vi "PCO_SetActiveRamSegment.vi"(8 "error in (no error)":errorcluster {"code" format="%x"}, 10 "wActSeg":u16, 11 "ph":u64) -> (0 "error out":errorcluster {"code" format="%x"}, 2 "ErrorMessage":i32 format="%x", 3 "ph out":u64)   [LabVIEW 2019, in "SDK.lvlib" / "StorageControl.lvlib"]
doc: "<b>Description:</b>\nThis function does set the active memory segment. Images from a subsequent recording are stored in the memory of the active segment. Relevant settings of the recorded images are also stored for each segment see also PCO_GetSegmentImageSettings.\nThis command will be rejected, if Recording State is [run], see PCO_GetRecordingState.\n\n<b>Supported camera type:</b>\npco.dimax, pco.1200, pco.1600, pco.2000, pco.4000\n\n<b>Descriptor dependency:</b>\ndwGeneralCapsDESC1: NO_RECORDER"
uses:
  StorageControl.lvlib
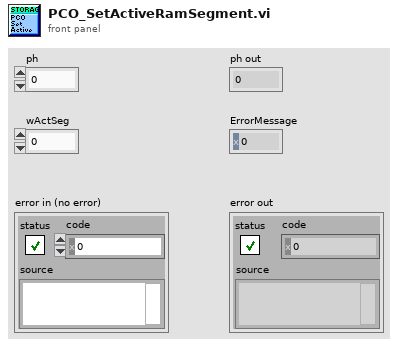
[diagram p1: front panel]
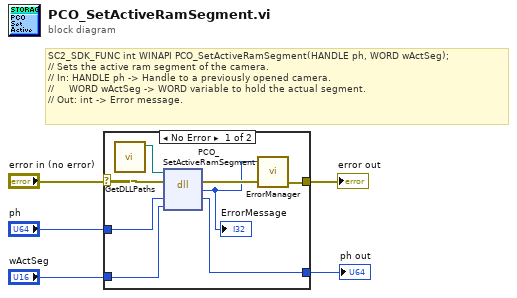
[diagram p0: block diagram]
diagram:
  # "SC2_SDK_FUNC int WINAPI PCO_SetActiveRamSegment(HANDLE ph, WORD wActSeg);\n// Sets the active ram segment of the camera.\n// In: HANDLE ph -> Handle to a previously opened camera.\n//     WORD wActSeg -> WORD variable to hold the actual segment.\n// Out: int -> Error message."
  n1 = case shown="No Error" "error in (no error)" {
    selector: "error in (no error)" -> [w10 w15]
    tunnel: "ph" -> [w13 w14]
    tunnel: [w12 w14] -> w4
    tunnel: "wActSeg" -> [w11 _]
    tunnel: [w8 w15] -> w2
    frame No Error {
      n2 = call "GetDLLPaths.vi"() -> ("SC2_Cam_Path"=w6:path)  [unwired: 8 in, 3 out]
      n3 = dll-call lib="?" fn="PCO_SetActiveRamSegment"(path in=w6, error in=w10, "ph"=w13, "wActSeg"=w11) -> (error out=w9:errorcluster, "return type"=w7:i32, "ph"=w12:u64)  [unwired: 2 in, 1 out]
      "ErrorMessage" <- w7
      n4 = call "ErrorManager.vi"("error in (no error)"=w9, "error code"=w7) -> ("error out"=w8:errorcluster)  [unwired: 2 in, 1 out]
    }
    frame Error {
    }
  }
  "ph out" <- w4
  "error out" <- w2
